vi "Get RHS.vi"(8 "error in (no error)":errorcluster, 10 "Domain":refnum<class "NI_Domain.lvclass">, 11 "RHS_3D_VIRef in":refnum<class "NI_RHS_3D_VIRef.lvclass">) -> (0 "error out":errorcluster, 2 "RHS":variant, 3 "RHS_3D_VIRef out":refnum<class "NI_RHS_3D_VIRef.lvclass">)   [LabVIEW 2020, in "NI_PDE.lvlib" / "NI_RHS_3D_VIRef.lvclass"]
uses:
  <vilib>/gmath/pde.llb/RHSClass/RHS_3D_VIRef/NI_RHS_3D_VIRef.lvclass
  <vilib>/gmath/pde.llb/DomainClass/NI_Domain.lvclass
  <vilib>/gmath/pde.llb/RHSClass/RHS_3D_VIRef/RHS Data.ctl
  <vilib>/gmath/pde.llb/RHSClass/RHS_3D_VIRef/NI_RHS_3D_VIRef.lvclass/NI_RHS_3D_VIRef.ctl
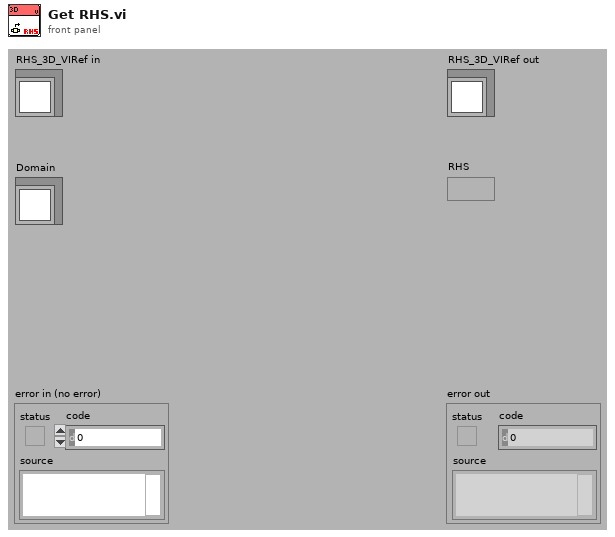
[diagram p1: front panel]
types:
  T1 = typedef "NI_PDE.lvlib/NI_RHS_3D_VIRef.lvclass/RHS Data.ctl" = cluster{"F":refnum<vi>, "data":variant}
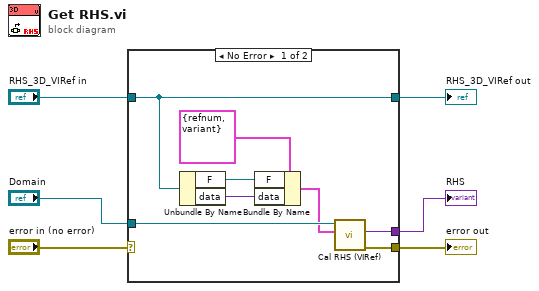
[diagram p0: block diagram]
diagram:
  n1 = case shown="No Error" "error in (no error)" {
    selector: "error in (no error)" -> [_ w15]
    tunnel: "RHS_3D_VIRef in" -> [w8 w16]
    tunnel: [w13 _] -> w5
    tunnel: [w8 w16] -> w4
    tunnel: [w12 w15] -> w3
    tunnel: "Domain" -> [w14 _]
    frame No Error {
      n2 = Unbundle By Name(w8) -> ("F"=w10:refnum<vi>, "data"=w9:variant)
      n3 = Bundle By Name(cluster=T1 {"F"=refnum, "data"=variant} ("RHS data"), "F"=w10, "data"=w9) -> (w7:T1)
      n4 = call-dynamic "Cal RHS (VIRef).vi"("RHS in"=w7, "Domain in"=w14) -> ("error out"=w12:errorcluster, "RHS out"=w13:variant)  [unwired: 1 in, 7 out]
    }
    frame Error {
    }
  }
  "RHS" <- w5
  "error out" <- w3
  "RHS_3D_VIRef out" <- w4
